vi "OutputToINI.vi"(5 "RStatus":string, 6 "Error":string, 7 "RValue":string, 8 "error in (no error)":errorcluster, 9 "Step Type":string, 10 "Step Name":string, 11 "Path":path) -> (0 "error out":errorcluster)   [LabVIEW 2015]
doc: "Use this template to build a VI to use as a subVI."
uses:
  <vilib>/Utility/config.llb/NI_LVConfig.lvlib
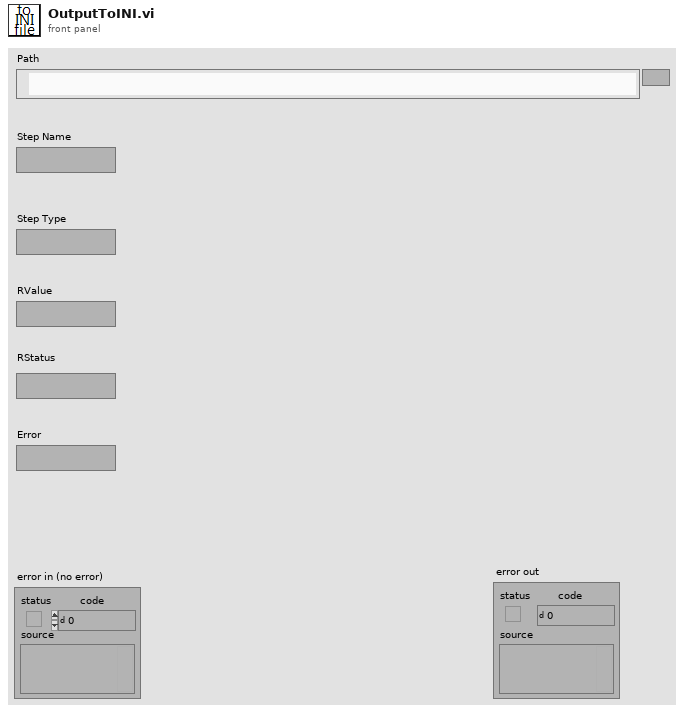
[diagram p1: front panel]
types:
  T1 = typedef "NI_LVConfig.lvlib/Config Data RefNum.ctl" = refnum<k1>
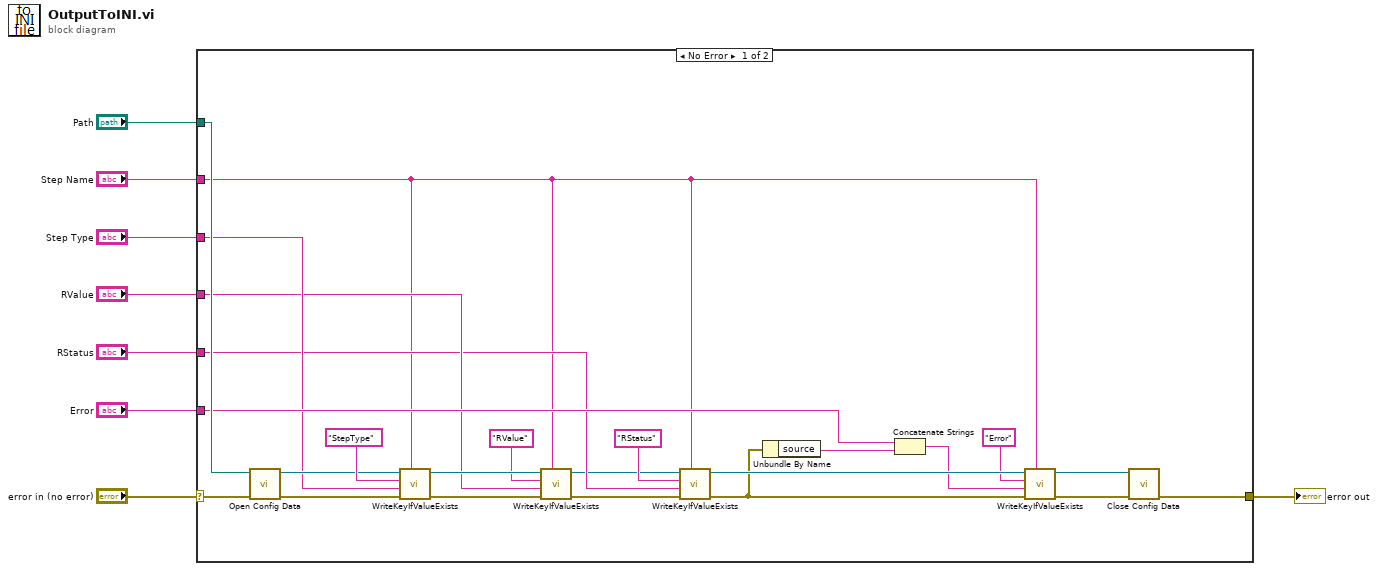
[diagram p0: block diagram]
diagram:
  n1 = case shown="No Error" "error in (no error)" {
    selector: "error in (no error)" -> [w32 w33]
    tunnel: [w31 w33] -> w7
    tunnel: "Path" -> [w30 _]
    tunnel: "Step Name" -> [w16 _]
    tunnel: "Step Type" -> [w26 _]
    tunnel: "RValue" -> [w22 _]
    tunnel: "RStatus" -> [w19 _]
    tunnel: "Error" -> [w29 _]
    frame No Error {
      n2 = call <vilib>:"Open Config Data.vi"("error in (no error)"=w32, "configuration file path"=w30) -> ("error out"=w25:errorcluster, "refnum"=w27:T1)  [unwired: 7 in, 1 out]
      n3 = call "WriteKeyIfValueExists.vi"("section"=w16, "error in (no error)"=w25, "value"=w26, "key"="StepType", "refnum out"=w27) -> ("error out"=w21:errorcluster, "refnum out"=w24:T1)  [unwired: 4 in, 1 out]
      n4 = call "WriteKeyIfValueExists.vi"("section"=w16, "error in (no error)"=w21, "value"=w22, "key"="RValue", "refnum out"=w24) -> ("error out"=w20:errorcluster, "refnum out"=w17:T1)  [unwired: 4 in, 1 out]
      n5 = call "WriteKeyIfValueExists.vi"("section"=w16, "error in (no error)"=w20, "value"=w19, "key"="RStatus", "refnum out"=w17) -> ("error out"=w11:errorcluster, "refnum out"=w14:T1)  [unwired: 4 in, 1 out]
      n6 = Unbundle By Name(w11) -> ("source"=w9:string)
      n7 = Concatenate Strings(w29, w9) -> (w12:string)
      n8 = call "WriteKeyIfValueExists.vi"("section"=w16, "error in (no error)"=w11, "value"=w12, "key"="Error", "refnum out"=w14) -> ("error out"=w10:errorcluster, "refnum out"=w15:T1)  [unwired: 4 in, 1 out]
      n9 = call <vilib>:"Close Config Data.vi"("error in (no error)"=w10, "refnum"=w15) -> ("error out"=w31:errorcluster)  [unwired: 8 in, 1 out]
    }
    frame Error {
    }
  }
  "error out" <- w7
